vi "Lex Numeric Number.vi"(8 "error in (no error)":errorcluster, 11 "JSON Lexer in":refnum<class "JSON Lexer.lvclass">) -> (0 "error out":errorcluster, 1 "EOF":bool, 2 "Next State":T1=enum."Value", 3 "JSON Lexer out":refnum<class "JSON Lexer.lvclass">)   [LabVIEW 2013, in "JKI JSON Serialization.lvlib" / "JSON Lexer.lvclass"]
uses:
  JSON Lexer.lvclass
  JSON Lexer States.ctl
  JSON Token Type.ctl
  JSON Lexer.lvclass/JSON Lexer.ctl
  <vilib>/addons/_JKI.lib/Unicode/UTF-8 String/UTF-8 String.lvclass/UTF-8 String.ctl
  Backup.vi
  Next.vi
  Ignore.vi
  <vilib>/addons/_JKI.lib/Unicode/UTF-8 String/Index Rune as UTF-8 Substring.vi
  <vilib>/addons/_JKI.lib/Unicode/UTF-8 String/Next Rune As UTF-8 Substring.vi
  <vilib>/addons/_JKI.lib/Unicode/UTF-8 String/Bytes In Rune.vi
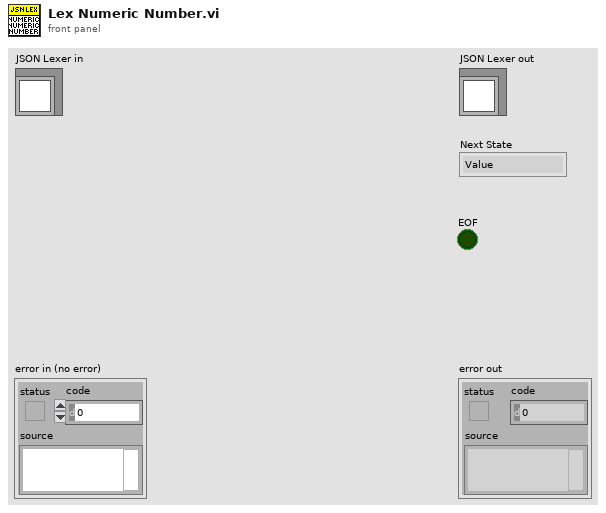
[diagram p1: front panel]
types:
  T1 = typedef "JKI JSON Serialization.lvlib/JSON Lexer.lvclass/JSON Lexer States.ctl" = enum16{"Undefined", "Value", "String", "Numeric", "Number", "Symbol", "Symbolic Number"}
  T2 = typedef "JKI JSON Serialization.lvlib/JSON Lexer.lvclass/JSON Token Type.ctl" = enum32{"unknown", "comma", "end-label", "begin-object", "end-object", "begin-array", "end-array", "quoted-string", "boolean", "exponential-number", "decimal-number", "integer-number", "special-number", "null", "symbol", "whitespace", "EOF"}
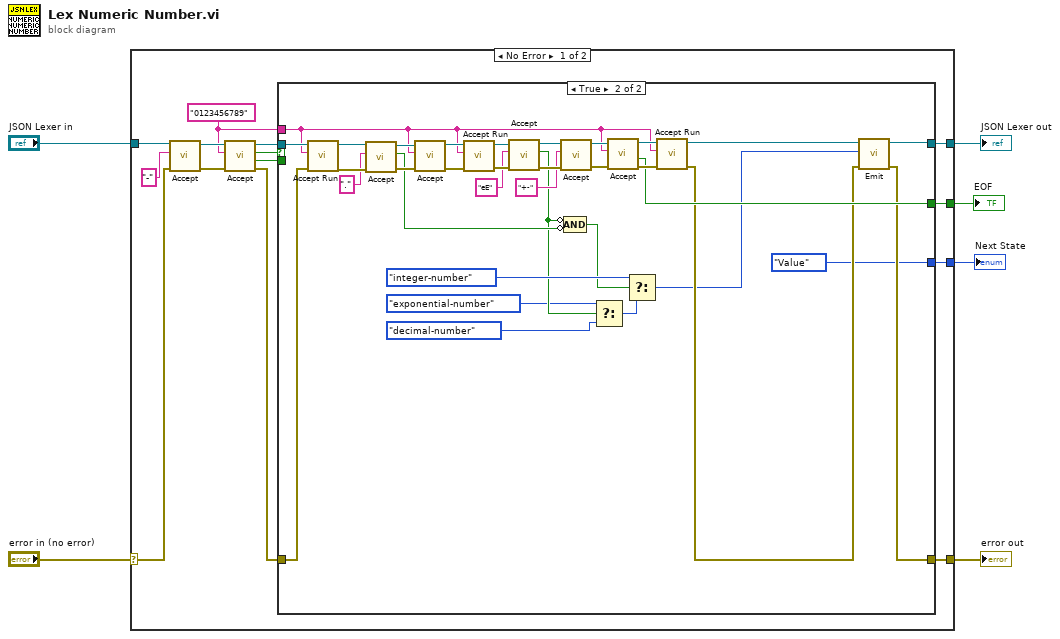
[diagram p0: block diagram]
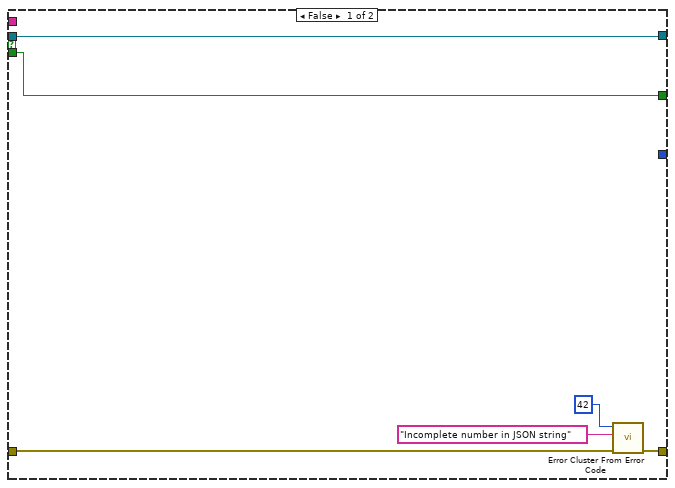
[diagram p2: hidden frame]
diagram:
  n1 = case shown="No Error" "error in (no error)" {
    selector: "error in (no error)" -> [w17 w62]
    tunnel: [w10 w62] -> w5
    tunnel: [w18 w61] -> w3
    tunnel: "JSON Lexer in" -> [w16 w61]
    tunnel: [w8 _] -> w2
    tunnel: [w7 _] -> w1
    frame No Error {
      w12 = "0123456789" ("Accepted Runes")
      n2 = call "Accept.vi"("error in (no error)"=w17, "Accepted Runes"="-", "JSON Lexer in"=w16) -> ("error out"=w19:errorcluster, "JSON Lexer out"=w20:refnum<class "JSON Lexer.lvclass">)  [unwired: 4 in, 3 out]
      n3 = call "Accept.vi"("error in (no error)"=w19, "Accepted Runes"=w12, "JSON Lexer in"=w20) -> ("error out"=w13:errorcluster, "EOF"=w9:bool, "Accepted?"=w11:bool, "JSON Lexer out"=w14:refnum<class "JSON Lexer.lvclass">)  [unwired: 4 in, 1 out]
      n4 = case shown="True" w11 {
        tunnel: [w21 w38] -> w18
        tunnel: w14 -> [w21 w60]
        tunnel: w13 -> [w25 w59]
        tunnel: w12 -> [_ w41]
        tunnel: [w26 w36] -> w10
        tunnel: w9 -> [w22 _]
        tunnel: [w22 w40] -> w8
        tunnel: [_ JSON_Lexer_States."Value" ("JSON Lexer State")] -> w7
        frame False {
          n5 = call <vilib>:"Error Cluster From Error Code.vi"("error in (no error)"=w25, "error message (\"\")"="Incomplete number in JSON string" ("error message (\"\")"), "error code (0)"=42) -> ("error out"=w26:errorcluster)  [unwired: 6 in]
        }
        frame True {
          n6 = call "Accept Run.vi"("error in (no error)"=w59, "Accepted Runes"=w41, "JSON Lexer in"=w60) -> ("error out"=w57:errorcluster, "JSON Lexer out"=w58:refnum<class "JSON Lexer.lvclass">)  [unwired: 7 in]
          n7 = call "Accept.vi"("error in (no error)"=w57, "Accepted Runes"=".", "JSON Lexer in"=w58) -> ("error out"=w54:errorcluster, "Accepted?"=w34:bool, "JSON Lexer out"=w55:refnum<class "JSON Lexer.lvclass">)  [unwired: 4 in, 2 out]
          n8 = call "Accept.vi"("error in (no error)"=w54, "Accepted Runes"=w41, "JSON Lexer in"=w55) -> ("error out"=w52:errorcluster, "JSON Lexer out"=w53:refnum<class "JSON Lexer.lvclass">)  [unwired: 4 in, 3 out]
          n9 = call "Accept Run.vi"("error in (no error)"=w52, "Accepted Runes"=w41, "JSON Lexer in"=w53) -> ("error out"=w50:errorcluster, "JSON Lexer out"=w51:refnum<class "JSON Lexer.lvclass">)  [unwired: 7 in]
          n10 = call "Accept.vi"("error in (no error)"=w50, "Accepted Runes"="eE", "JSON Lexer in"=w51) -> ("error out"=w47:errorcluster, "Accepted?"=w31:bool, "JSON Lexer out"=w48:refnum<class "JSON Lexer.lvclass">)  [unwired: 4 in, 2 out]
          n11 = call "Accept.vi"("error in (no error)"=w47, "Accepted Runes"="+-", "JSON Lexer in"=w48) -> ("error out"=w44:errorcluster, "JSON Lexer out"=w45:refnum<class "JSON Lexer.lvclass">)  [unwired: 4 in, 3 out]
          n12 = Compound Arithmetic op=AND(invert w31, invert w34) -> (w32:bool)
          n13 = Select(t=JSON_Token_Type."exponential-number" ("JSON Token Type"), s=w31, f=JSON_Token_Type."decimal-number" ("JSON Token Type")) -> (s? t:f=w28:T2)
          n14 = call "Accept.vi"("error in (no error)"=w44, "Accepted Runes"=w41, "JSON Lexer in"=w45) -> ("error out"=w42:errorcluster, "EOF"=w40:bool, "JSON Lexer out"=w43:refnum<class "JSON Lexer.lvclass">)  [unwired: 4 in, 2 out]
          n15 = Select(t=JSON_Token_Type."integer-number" ("JSON Token Type"), s=w32, f=w28) -> (s? t:f=w27:T2)
          n16 = call "Accept Run.vi"("error in (no error)"=w42, "Accepted Runes"=w41, "JSON Lexer in"=w43) -> ("error out"=w37:errorcluster, "JSON Lexer out"=w39:refnum<class "JSON Lexer.lvclass">)  [unwired: 7 in]
          n17 = call "Emit.vi"("error in (no error)"=w37, "JSON Token Type"=w27, "JSON Lexer in"=w39) -> ("error out"=w36:errorcluster, "JSON Lexer out"=w38:refnum<class "JSON Lexer.lvclass">)  [unwired: 7 in]
        }
      }
    }
    frame Error {
    }
  }
  "error out" <- w5
  "JSON Lexer out" <- w3
  "Next State" <- w1
  "EOF" <- w2
